vi "Update Setting.vi"(6 "Update Setting:":T1, 8 "error in":errorcluster, 11 "IMG_SRC in":refnum<class "IMG_SRC.lvclass">) -> (0 "error out":errorcluster, 2 "Supported?":bool, 3 "IMG_SRC out":refnum<class "IMG_SRC.lvclass">)   [LabVIEW 2018, in "IMG_SRC.lvlib" / "IMG_SRC.lvclass"]
uses:
  IMG_SRC.lvclass
  builds/Camera.lvlibp/Custom Controls/Camera Setting.ctl
  builds/Camera.lvlibp/Camera.lvclass
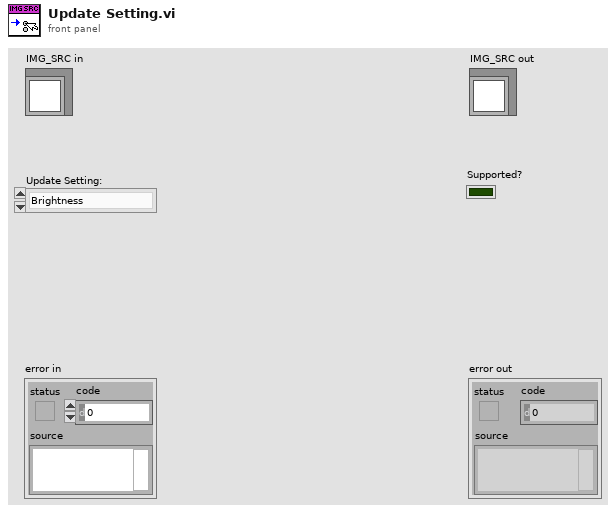
[diagram p1: front panel]
types:
  T1 = typedef "Camera.lvlibp/Camera.lvclass/Camera Setting.ctl" = enum16{"Brightness", "Rotation", "Contrast", "Exposure", "Frame Rate", "Gain", "Gamma", "Image Resolution", "Sharpness"}
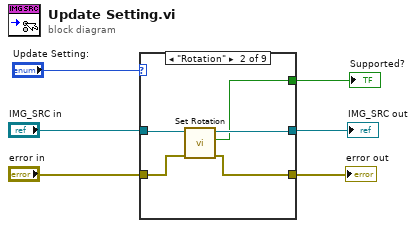
[diagram p0: block diagram]
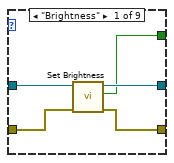
[diagram p2: hidden frame]
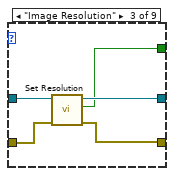
[diagram p3: hidden frame]
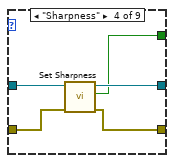
[diagram p4: hidden frame]
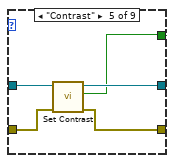
[diagram p5: hidden frame]
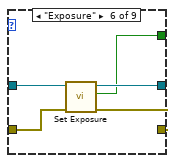
[diagram p6: hidden frame]
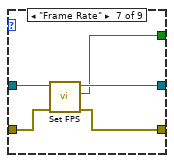
[diagram p7: hidden frame]
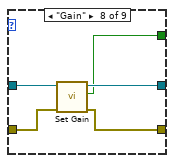
[diagram p8: hidden frame]
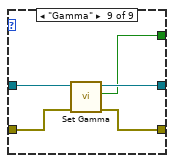
[diagram p9: hidden frame]
diagram:
  n1 = case shown="\"Rotation\"" "Update Setting:" {
    tunnel: "IMG_SRC in" -> [w11 w16 w21 w25 w30 w35 w41 w46 w51]
    tunnel: "error in" -> [w10 w15 w20 w26 w31 w36 w40 w45 w49]
    tunnel: [w9 w13 w18 w24 w28 w33 w38 w43 w48] -> w1
    tunnel: [w8 w14 w19 w23 w29 w34 w39 w44 w50] -> w2
    tunnel: [w7 w12 w17 w22 w27 w32 w37 w42 w47] -> w5
    frame "Brightness" {
      n2 = call "Set Brightness.vi"("error in"=w10, "IMG_SRC in"=w11) -> ("error out"=w9:errorcluster, "Supported?"=w7:bool, "IMG_SRC out"=w8:refnum<class "IMG_SRC.lvclass">)  [unwired: 7 in]
    }
    frame "Rotation" {
      n3 = call "Set Rotation.vi"("error in"=w15, "IMG_SRC in"=w16) -> ("error out"=w13:errorcluster, "Supported?"=w12:bool, "IMG_SRC out"=w14:refnum<class "IMG_SRC.lvclass">)  [unwired: 7 in]
    }
    frame "Image Resolution" {
      n4 = call "Set Resolution.vi"("error in"=w20, "IMG_SRC in"=w21) -> ("error out"=w18:errorcluster, "Supported?"=w17:bool, "IMG_SRC out"=w19:refnum<class "IMG_SRC.lvclass">)  [unwired: 7 in]
    }
    frame "Sharpness" {
      n5 = call "Set Sharpness.vi"("error in"=w26, "IMG_SRC in"=w25) -> ("error out"=w24:errorcluster, "Supported?"=w22:bool, "IMG_SRC out"=w23:refnum<class "IMG_SRC.lvclass">)  [unwired: 7 in]
    }
    frame "Contrast" {
      n6 = call "Set Contrast.vi"("error in"=w31, "IMG_SRC in"=w30) -> ("error out"=w28:errorcluster, "Supported?"=w27:bool, "IMG_SRC out"=w29:refnum<class "IMG_SRC.lvclass">)  [unwired: 7 in]
    }
    frame "Exposure" {
      n7 = call "Set Exposure.vi"("error in"=w36, "IMG_SRC in"=w35) -> ("error out"=w33:errorcluster, "Supported?"=w32:bool, "IMG_SRC out"=w34:refnum<class "IMG_SRC.lvclass">)  [unwired: 7 in]
    }
    frame "Frame Rate" {
      n8 = call "Set FPS.vi"("error in"=w40, "IMG_SRC in"=w41) -> ("error out"=w38:errorcluster, "Supported?"=w37:bool, "IMG_SRC out"=w39:refnum<class "IMG_SRC.lvclass">)  [unwired: 7 in]
    }
    frame "Gain" {
      n9 = call "Set Gain.vi"("error in"=w45, "IMG_SRC in"=w46) -> ("error out"=w43:errorcluster, "Supported?"=w42:bool, "IMG_SRC out"=w44:refnum<class "IMG_SRC.lvclass">)  [unwired: 7 in]
    }
    frame "Gamma" {
      n10 = call "Set Gamma.vi"("error in"=w49, "IMG_SRC in"=w51) -> ("error out"=w48:errorcluster, "Supported?"=w47:bool, "IMG_SRC out"=w50:refnum<class "IMG_SRC.lvclass">)  [unwired: 7 in]
    }
  }
  "error out" <- w1
  "IMG_SRC out" <- w2
  "Supported?" <- w5
